vi "Initialize Osciloscope.vi"(8 "error in (no error)":errorcluster, 10 "Initialize--cluster":T1={"TEKTRONIX-INITIALIZE"={"ID Query? (T: Yes)"=TRUE, "Reset? (T: Yes)"=TRUE, "Serial-Configuration"={"Baud Rate"=9600, "Parity"=0, "Stop Bits"=10, "Flow Control"=2}}, "EDU-X-1200A- INITIALIZE"={"Reset (True)"=TRUE, "ID Query (True)"=TRUE}} {"TEKTRONIX-INITIALIZE"."Serial-Configuration"."Flow Control" items=["None", "XON/XOFF", "RTS/CTS", "XON/XOFF & RTS/CTS", "DTR/DSR", "XON/XOFF & DTR/DSR"]; "TEKTRONIX-INITIALIZE"."Serial-Configuration"."Stop Bits" items=["1.0"=10, "1.5"=15, "2.0"=20]; "TEKTRONIX-INITIALIZE"."Serial-Configuration"."Parity" items=["None", "Odd", "Even", "Mark", "Space"]; "TEKTRONIX-INITIALIZE"."Serial-Configuration"."Baud Rate" items=["300"=300, "600"=600, "1200"=1200, "2400"=2400, "4800"=4800, "9600"=9600, "19200"=19200]}, 11 "OsciloscopeClass in":refnum<class "OsciloscopeClass.lvclass">) -> (0 "error out":errorcluster, 3 "OsciloscopeClass out":refnum<class "OsciloscopeClass.lvclass">)   [LabVIEW 2020, in "OsciloscopeClass.lvclass"]
uses:
  OsciloscopeClass.lvclass
  TypeDefs/InitializeOsciloscope--cluster.ctl
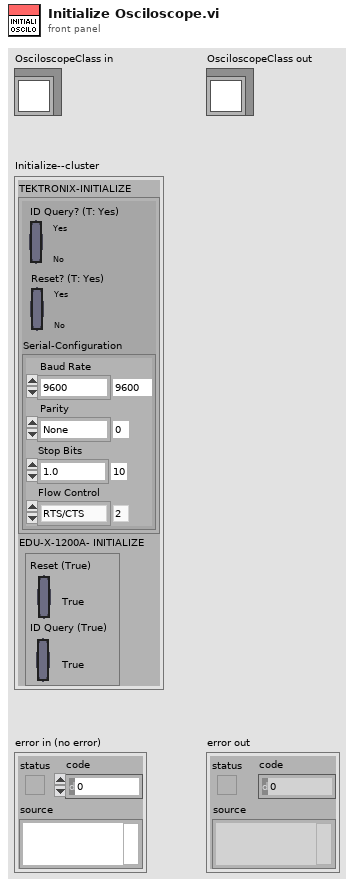
[diagram p1: front panel]
types:
  T1 = typedef "InitializeOsciloscope--cluster.ctl" = cluster{"TEKTRONIX-INITIALIZE":cluster{"ID Query? (T: Yes)":bool, "Reset? (T: Yes)":bool, "Serial-Configuration":cluster{"Baud Rate":u32, "Parity":u16, "Stop Bits":u16, "Flow Control":u16}}, "EDU-X-1200A- INITIALIZE":cluster{"Reset (True)":bool, "ID Query (True)":bool}}
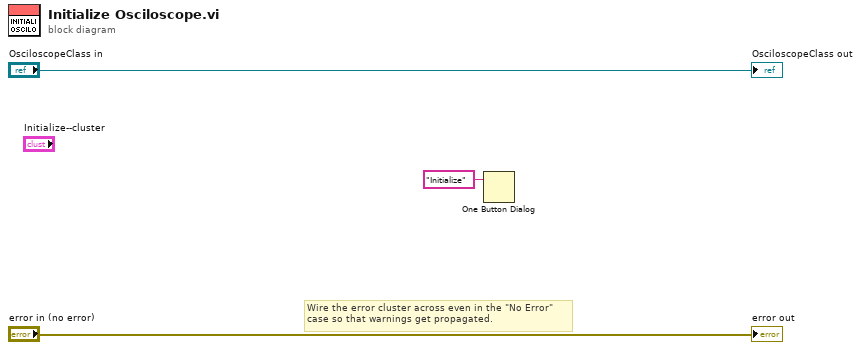
[diagram p0: block diagram]
diagram:
  # "Wire the error cluster across even in the \"No Error\"\ncase so that warnings get propagated."
  n1 = One Button Dialog(message="Initialize") -> ()  [unwired: 1 in, 1 out]
  "error out" <- "error in (no error)"
  "OsciloscopeClass out" <- "OsciloscopeClass in"
